vi "HandleSelect.vi"(8 "error in (no error)":errorcluster, 11 "Menu in":refnum<class "Menu.lvclass">) -> (0 "error out":errorcluster, 3 "Menu out":refnum<class "Menu.lvclass">)   [LabVIEW 2019, in "RT_Game.lvlib" / "Menu.lvclass"]
uses:
  Menu.lvclass
  C:/Users/FreshBob/Dropbox/VIs/myRIO_GameConsole/RT/RT_Game/Game/Game.lvclass
  Game/Game.lvclass/Game.ctl
  Game/Game.lvclass
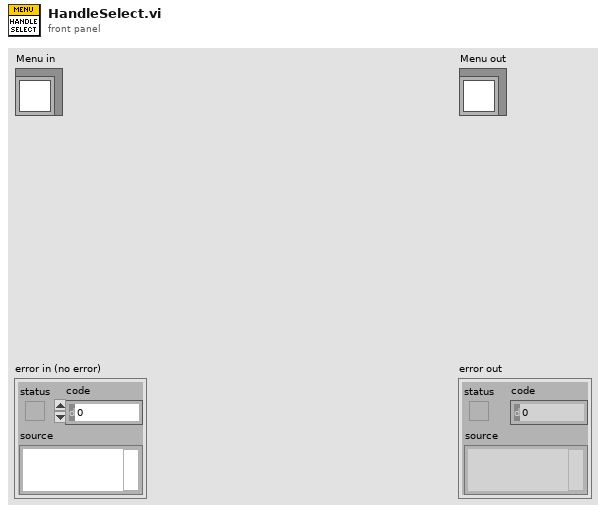
[diagram p1: front panel]
types:
  T1 = cluster{"Controls_1":cluster{"DirectionX":i8, "DirectionY":i8, "Button1":bool, "Button2":bool}, "Controls_2":cluster{"DirectionX":i8, "DirectionY":i8, "Button1":bool, "Button2":bool}, "SystemButton":bool}
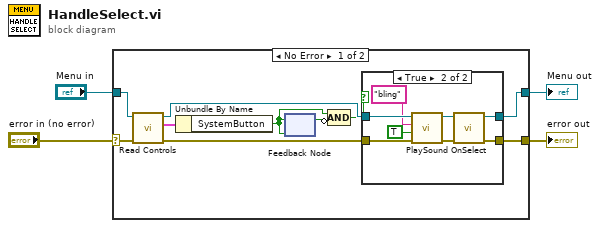
[diagram p0: block diagram]
diagram:
  n1 = case shown="No Error" "error in (no error)" {
    selector: "error in (no error)" -> [w14 w26]
    tunnel: [w8 w26] -> w3
    tunnel: [w6 w25] -> w1
    tunnel: "Menu in" -> [w12 w25]
    frame No Error {
      n2 = call "Read Controls.vi"("error in (no error)"=w14, "Game in"=w12) -> ("error out"=w13:errorcluster, "Controls"=w11:T1, "Game out"=w7:refnum<class "Menu.lvclass">)  [unwired: 7 in]
      n3 = Unbundle By Name(w11) -> ("SystemButton"=w10:bool)
      n4 = feedback-in #1(w10) -> ()
      n5 = feedback #1(w10) -> (w9:bool)
      n6 = Compound Arithmetic op=AND(w10, invert w9) -> (w5:bool)
      n7 = case shown="True" w5 {
        tunnel: w13 -> [w15 w24]
        tunnel: [w15 w23] -> w8
        tunnel: w7 -> [w16 w20]
        tunnel: [w16 w22] -> w6
        frame False {
        }
        frame True {
          n8 = call "PlaySound.vi"("error in (no error)"=w24, "Overwrite"=TRUE, "Name"="bling", "Game in"=w20) -> ("error out"=w21:errorcluster, "Game out"=w19:refnum<class "Menu.lvclass">)  [unwired: 6 in]
          n9 = call-dynamic "OnSelect.vi"("error in (no error)"=w21, "Menu in"=w19) -> ("error out"=w23:errorcluster, "Menu out"=w22:refnum<class "Menu.lvclass">)  [unwired: 8 in]
        }
      }
    }
    frame Error {
    }
  }
  "error out" <- w3
  "Menu out" <- w1
